vi "EZ Freq and Period.vi"(6 "Freq/Period (F:Freq)":bool, 7 "Scan List (empty)":string, 8 "error in (no error)":errorcluster, 9 "Range (5:Auto)":u16(ring)=5 items=["100 mV", "1 V", "10 V", "100 V", "300 V", "Auto", "Minimum", "Maximum"], 10 "Low Frequency (1: 20 Hz)":u16(ring)=1 items=["3 Hz", "20 Hz", "200 Hz", "MIN", "MAX"], 11 "VISA Resource Name":refnum<visa-resource-name>) -> (0 "error out":errorcluster, 2 "Output Array":dbl[](array[numeric]) format="%.2f", 3 "VISA Resource Name Out":refnum<visa-resource-name>)   [LabVIEW 2012, in "Agilent 34970.lvlib"]
doc: "This VI lets you take simple frequency/period measurements."
uses:
  <instrlib>/Agilent 34970/Agilent 34970.lvlib
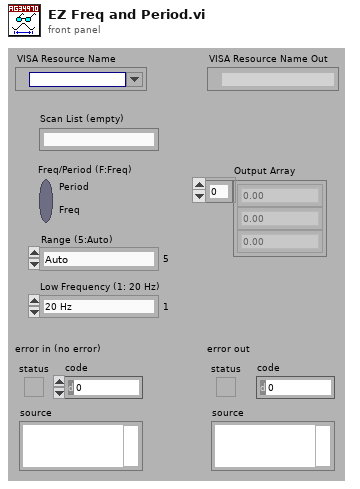
[diagram p1: front panel]
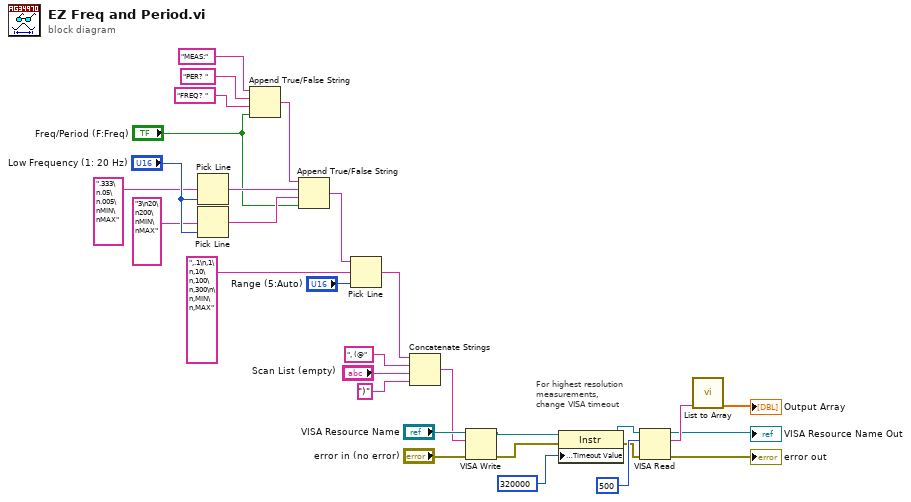
[diagram p0: block diagram]
diagram:
  # "For highest resolution\nmeasurements, \nchange VISA timeout"
  n1 = Pick Line(multi-line string=".333\n.05\n.005\nMIN\nMAX", line index="Low Frequency (1: 20 Hz)") -> (output string=w11:string)  [unwired: 1 in]
  n2 = Pick Line(multi-line string="3\n20\n200\nMIN\nMAX", line index="Low Frequency (1: 20 Hz)") -> (output string=w10:string)  [unwired: 1 in]
  n3 = Append True/False String(1:"Freq/Period (F:Freq)", 2:"FREQ? ", 3:"PER? ", 4:"MEAS:") -> (0:w9:string)
  n4 = Append True/False String(1:"Freq/Period (F:Freq)", 2:w10, 3:w11, 4:w9) -> (0:w7:string)
  n5 = Pick Line(string ("")=w7, multi-line string=",.1\n,1\n,10\n,100\n,300\n\n,MIN\n,MAX", line index="Range (5:Auto)") -> (output string=w6:string)
  n6 = Concatenate Strings(w6, ", (@", "Scan List (empty)", ")") -> (w15:string)
  n7 = VISA Write(VISA resource name="VISA Resource Name", write buffer=w15, error in (no error)="error in (no error)") -> (VISA resource name out=w4:refnum<visa-resource-name>, error out=w3:errorcluster)  [unwired: 1 out]
  n8 = property class="Instr"(reference=w4, error in=w3, "General Settings:Timeout Value"=u32 320000 ("Tmo Value")) -> (reference out=w2:refnum<visa-resource-name>, error out=w1:errorcluster)
  n9 = VISA Read(VISA resource name=w2, byte count=u32 500 ("byte count (0)"), error in (no error)=w1) -> (VISA resource name out=→"VISA Resource Name Out":refnum<visa-resource-name>, read buffer=w22:string, error out=→"error out":errorcluster)  [unwired: 1 out]
  n10 = call <instrlib>:"List to Array.vi"("List (empty)"=w22) -> ("Output Number Array"=→"Output Array":dbl[])  [unwired: 9 in, 1 out]
